vi "setCurrentLimit.vi"(8 "error in (no error)":errorcluster, 9 "Current Limit in A":dbl=10.0 format="%#_13g", 10 "Channel Nr (1)":string="1", 11 "VISA resource name":refnum<visa-resource-name>) -> (0 "error out":errorcluster, 3 "VISA resource name out":refnum<visa-resource-name>)   [LabVIEW 2023, in "Tti-Pl303Qmd.lvlib"]
doc: "Set Current Limit of Channel"
uses:
  Tti-Pl303Qmd.lvlib
  <vilib>/Utility/error.llb/Error Cluster From Error Code.vi
  <vilib>/ErrorRing/Error Ring.xnode
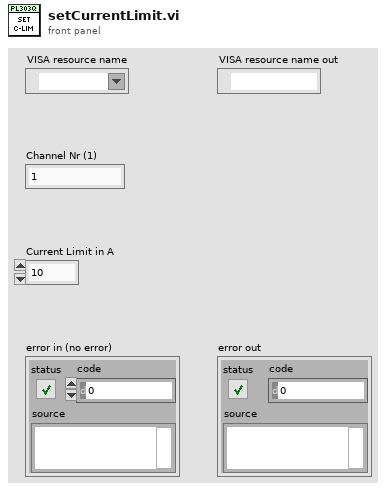
[diagram p1: front panel]
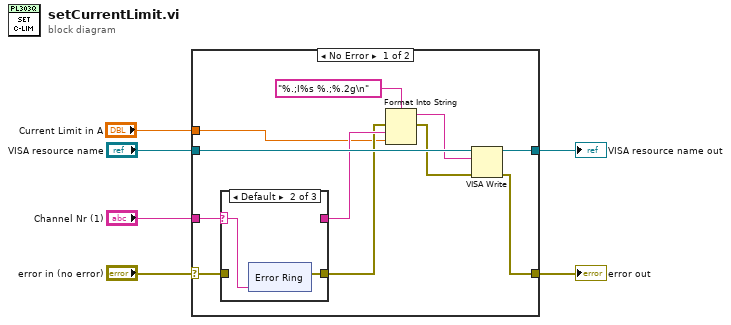
[diagram p0: block diagram]
diagram:
  n1 = case shown="No Error" "error in (no error)" {
    selector: "error in (no error)" -> [w14 w32]
    tunnel: "VISA resource name" -> [w16 w31]
    tunnel: [w17 w32] -> w6
    tunnel: "Channel Nr (1)" -> [w15 _]
    tunnel: "Current Limit in A" -> [w7 _]
    tunnel: [w8 w31] -> w1
    frame No Error {
      n2 = case shown="Default" w15 {
        selector: w15 -> [w19 w20 w29]
        tunnel: w14 -> [w18 _ w30]
        tunnel: [w18 w21 w30] -> w11
        tunnel: [w19 _ w29] -> w12
        frame "2" {
        }
        frame Default {
          n3 = xnode "Error Ring"("parameter 0"=w20) -> ("error out"=w21:errorcluster)
        }
        frame "1" {
        }
      }
      n4 = Format Into String(format string="%.;I%s %.;%.2g\n" ("write buffer"), error in=w11, w12, w7) -> (resulting string=w9:string, error out=w10:errorcluster)  [unwired: 1 in]
      n5 = VISA Write(VISA resource name=w16, write buffer=w9, error in (no error)=w10) -> (VISA resource name out=w8:refnum<visa-resource-name>, error out=w17:errorcluster)  [unwired: 1 out]
    }
    frame Error {
    }
  }
  "error out" <- w6
  "VISA resource name out" <- w1
